vi "Alternate Hierarchy.vi"() -> ()   [LabVIEW 2020]
uses:
  TSnax/Engine/Engine.lvclass
panel:
  out "Boolean":bool
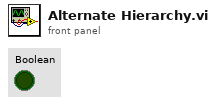
[diagram p1: front panel]
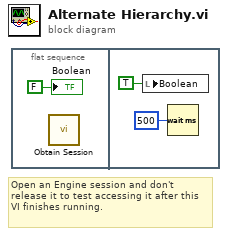
[diagram p0: block diagram]
diagram:
  # "Open an Engine session and don't release it to test accessing it after this VI finishes running."
  n1 = flat-sequence {
    frame #0 {
      n2 = call "Obtain Session.vi"() -> ()  [unwired: 10 in, 2 out]
      "Boolean" <- FALSE ("Boolean")
    }
    frame #1 {
      n3 = local write "Boolean"(TRUE ("Boolean")) -> ()
      n4 = Wait (ms)(milliseconds to wait=u32 500) -> ()  [unwired: 1 out]
    }
  }
